vi "Obtain Status.vi"(8 "error in (no error)":errorcluster, 11 "Input in":refnum<class "Input.lvclass">) -> (0 "error out":errorcluster, 1 "Status":string, 2 "Page":T1(ring), 3 "Input out":refnum<class "Input.lvclass">)   [LabVIEW 2023, in "Input.lvclass"]
uses:
  Input.lvclass
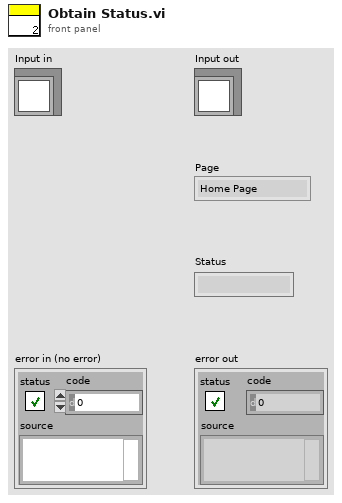
[diagram p1: front panel]
types:
  T1 = enum32{"Home Page", "Mode Page", "Configuration Page", "Input Page", "Result Page"}
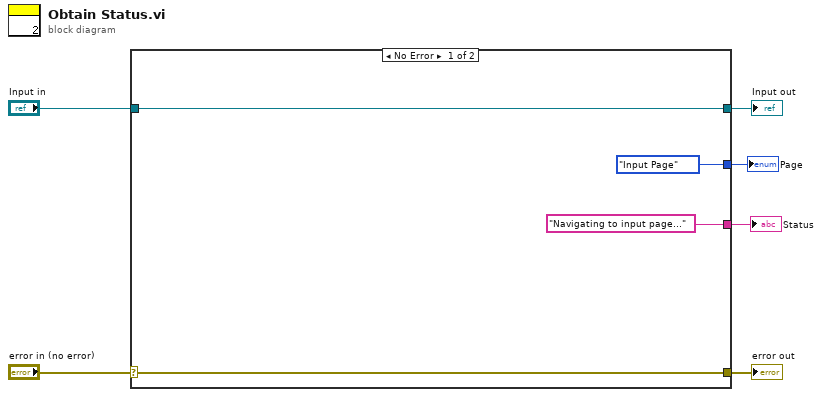
[diagram p0: block diagram]
diagram:
  n1 = case shown="No Error" "error in (no error)" {
    selector: "error in (no error)" -> [w9 w12]
    tunnel: [w9 w12] -> w5
    tunnel: [w10 w11] -> w3
    tunnel: "Input in" -> [w10 w11]
    tunnel: [T1."Input Page" ("Page") _] -> w2
    tunnel: ["Navigating to input page..." ("String") _] -> w1
    frame No Error {
    }
    frame Error {
    }
  }
  "error out" <- w5
  "Input out" <- w3
  "Page" <- w2
  "Status" <- w1
